vi "Write States.vi"(8 "error in (no error)":errorcluster, 10 "States":T1, 11 "GoToBallPlacementAllyTactic in":refnum<class "GoToBallPlacementAllyTactic.lvclass">) -> (0 "error out":errorcluster, 3 "GoToBallPlacementAllyTactic out":refnum<class "GoToBallPlacementAllyTactic.lvclass">)   [LabVIEW 2021, in "GoToBallPlacementAllyTactic.lvclass"]
uses:
  GoToBallPlacementAllyTactic.lvclass
  StatesGoToBallPlacementAllyTactic.ctl
  GoToBallPlacementAllyTactic.lvclass/GoToBallPlacementAllyTactic.ctl
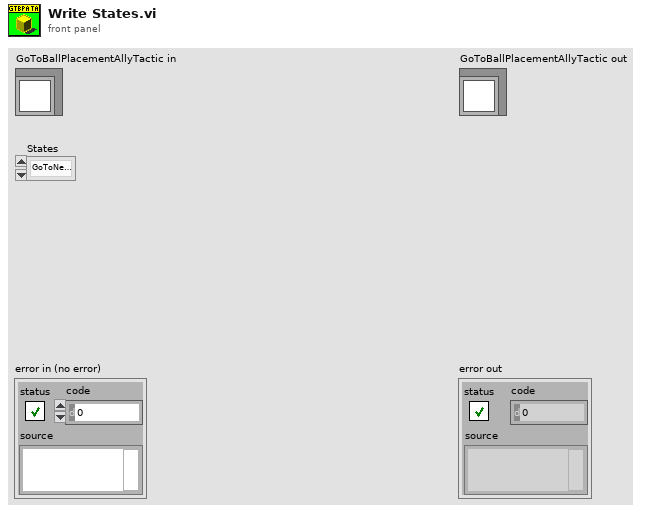
[diagram p1: front panel]
types:
  T1 = typedef "StatesGoToBallPlacementAllyTactic.ctl" = enum16{"GoToNearBall", "GoToBall", "PrepareToPositionBall", "Exit"}
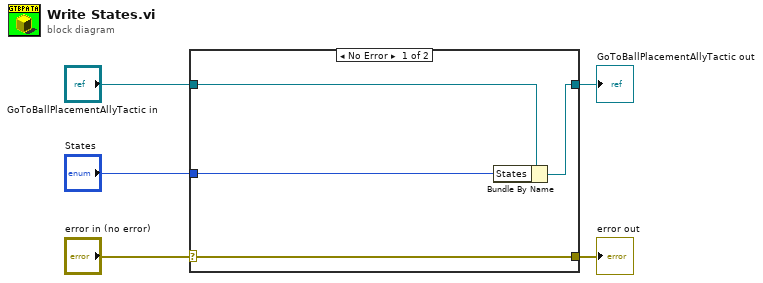
[diagram p0: block diagram]
diagram:
  n1 = case shown="No Error" "error in (no error)" {
    selector: "error in (no error)" -> [w9 w10]
    tunnel: [w9 w10] -> w4
    tunnel: [w7 w11] -> w2
    tunnel: "GoToBallPlacementAllyTactic in" -> [w8 w11]
    tunnel: "States" -> [w6 _]
    frame No Error {
      n2 = Bundle By Name(cluster=w8, "States"=w6) -> (w7:refnum<class "GoToBallPlacementAllyTactic.lvclass">)
    }
    frame Error {
    }
  }
  "error out" <- w4
  "GoToBallPlacementAllyTactic out" <- w2
